vi "Problem 5.vi"() -> ()   [LabVIEW 2025]
panel:
  out "Time to Run:":dbl
  out "Smallest number evenly divisble by all numbers from 1 to 20":i32
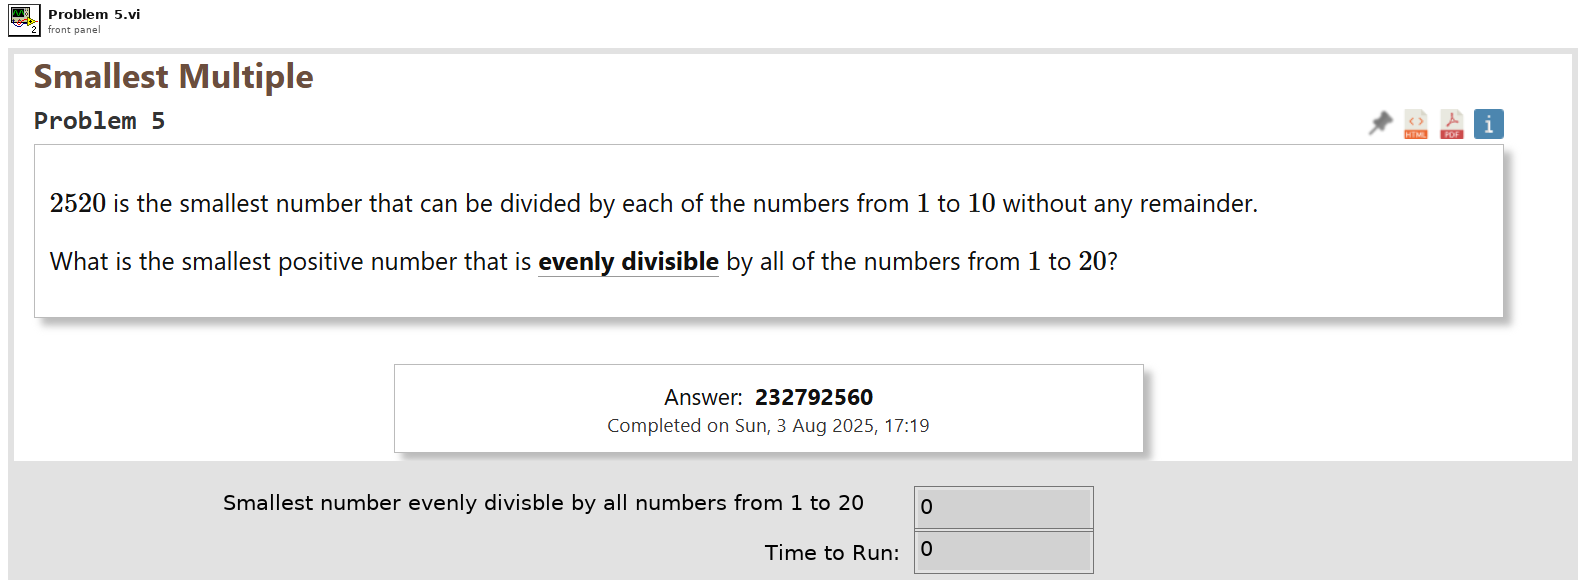
[diagram p1: front panel]
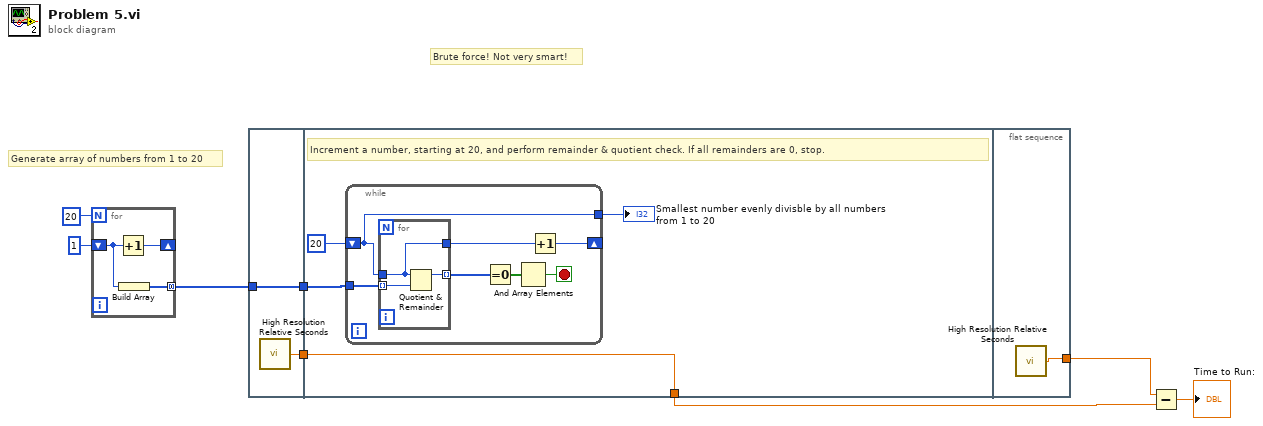
[diagram p0: block diagram]
diagram:
  # "Brute force! Not very smart!"
  # "Generate array of numbers from 1 to 20"
  n1 = for {
    N: 20 -> [_]
    tunnel: [w11] -> w6 mode=concatenating
    shift-right: [w9] -> _
    shift-left: 1 -> [w10]
    n2 = Increment(x=w10) -> (x+1=w9:i32)
    n3 = Build Array(w10) -> (w11:i32[])
  }
  n4 = flat-sequence {
    tunnel: w6 -> [w13]
    tunnel: [w13] -> w5
    tunnel: [w12] -> w4
    tunnel: w5 -> [w17]
    tunnel: w4 -> [w14]
    tunnel: [w14] -> w3
    tunnel: [w28] -> w2
    frame #0 {
      n5 = call <vilib>:"High Resolution Relative Seconds.vi"() -> ("relative seconds"=w12:dbl)
    }
    frame #1 {
      # "Increment a number, starting at 20, and perform remainder & quotient check. If all remainders are 0, stop."
      n6 = while {
        tunnel: w17 -> [w24]
        shift-right: [w20] -> _
        shift-left: 20 -> [w18]
        tunnel: [w18] -> w15
        stop <- w21 stop-if-true
        n7 = for {
          tunnel: w24 -> [w27] mode=indexing
          tunnel: [w26] -> w23 mode=indexing
          tunnel: w18 -> [w25]
          tunnel: [w25] -> w19
          n8 = Quotient & Remainder(x=w25, y=w27) -> (x-y*floor(x/y)=w26:i32)  [unwired: 1 out]
        }
        n9 = Equal To 0?(x=w23) -> (x = 0?=w22:bool[])
        n10 = And Array Elements(Boolean array=w22) -> (logical AND=w21:bool)
        n11 = Increment(x=w19) -> (x+1=w20:i32)
      }
      "Smallest number evenly divisble by all numbers from 1 to 20" <- w15
    }
    frame #2 {
      n12 = call <vilib>:"High Resolution Relative Seconds.vi"() -> ("relative seconds"=w28:dbl)
    }
  }
  n13 = Subtract(x=w2, y=w3) -> (x-y=→"Time to Run:":dbl)
